vi "Connect.vi"(4 "IP Address":string, 5 "error in (no error)":errorcluster, 6 "Camera Reference in":refnum<k24>) -> (0 "Result":bool, 1 "error out":errorcluster, 2 "Camera Reference out":refnum<k24>)   [LabVIEW 2023]
uses:
  C:/Program Files/National Instruments/LabVIEW 2025/MechEyeApiNet.dll
  Program Files/National Instruments/LabVIEW 2025/MechEyeApiNet.dll
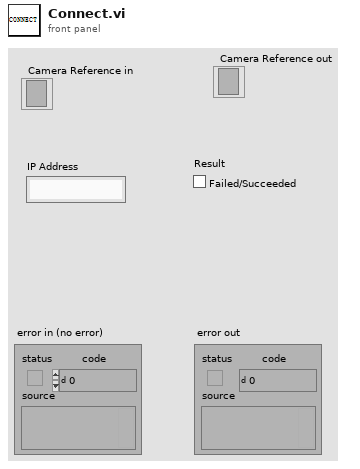
[diagram p1: front panel]
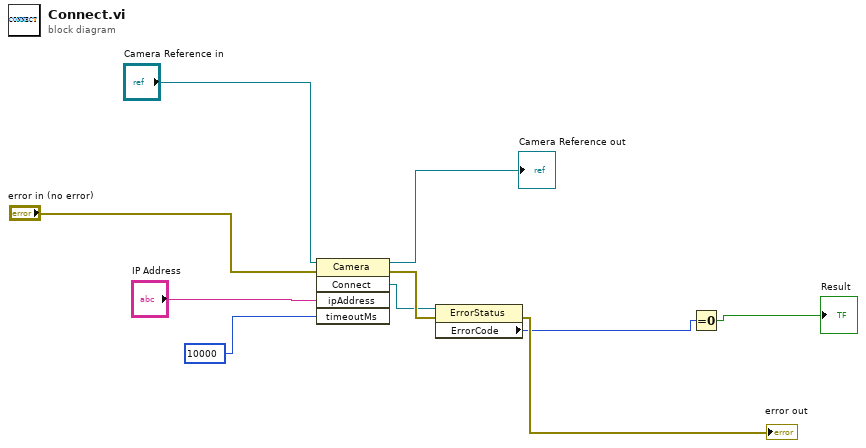
[diagram p0: block diagram]
diagram:
  n1 = invoke class="Camera" method="Connect"(reference="Camera Reference in", error in="error in (no error)", "ipAddress"="IP Address", "timeoutMs"=10000) -> (reference out=→"Camera Reference out":refnum<k24>, error out=w9:errorcluster, "Connect"=w3:refnum<k24>)  [unwired: 1 in, 2 out]
  n2 = property class="ErrorStatus"(reference=w3, error in=w9) -> (error out=→"error out":errorcluster, "ErrorCode"=w4:i32)  [unwired: 1 out]
  n3 = Equal To 0?(x=w4) -> (x = 0?=→"Result":bool)
